vi "Launch View.vi"(8 "error in (no error)":errorcluster, 10 "ConsoleView in":refnum<class "ConsoleView.lvclass">, 11 "ConsoleInterface in":refnum<class "ConsoleSession.lvclass">) -> (0 "error out":errorcluster, 3 "ConsoleInterface out":refnum<class "ConsoleSession.lvclass">)   [LabVIEW 2019, in "ConsoleView.lvlib" / "ConsoleSession.lvclass"]
uses:
  <vilib>/gpm_packages/@cs/event-logger/Source/ConsoleView/ConsoleInterface/ConsoleSession.lvclass
  <vilib>/gpm_packages/@cs/event-logger/Source/ConsoleView/View/ConsoleView.lvclass
  <vilib>/gpm_packages/@cs/event-logger/Source/Composed Log/Types/MessageCluster.ctl
  <vilib>/gpm_packages/@cs/event-logger/Source/ConsoleView/ConsoleInterface/ConsoleSession.lvclass/ConsoleSession.ctl
  <vilib>/gpm_packages/@cs/event-logger/Source/Composed Log/Composed Log.lvlib
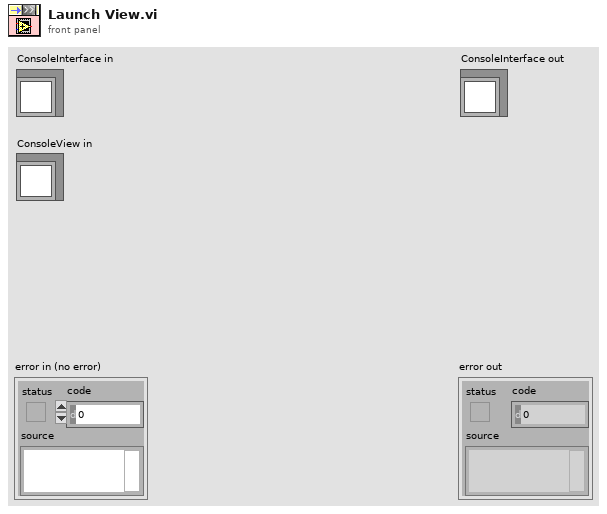
[diagram p1: front panel]
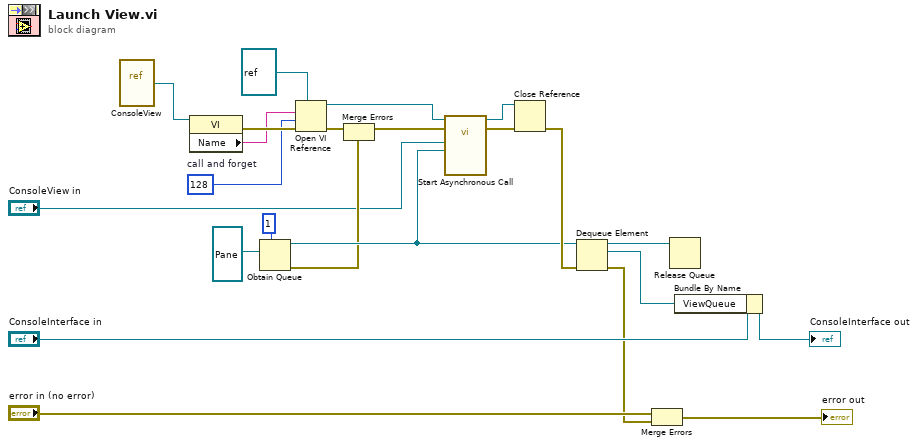
[diagram p0: block diagram]
diagram:
  w19 = 128  # call and forget
  n1 = vi-ref <vilib>:"ConsoleView.vi"() -> (w21:refnum<vi>)
  n2 = property class="VI"(reference=w21) -> (error out=w20:errorcluster, "Name"=w18:string)  [unwired: 1 in, 1 out]
  n3 = Obtain Queue(max queue size (-1, unlimited)=1, element data type=refnum<queue> refnum ("queue out")) -> (queue out=w13:refnum<queue>, error out=w10:errorcluster)  [unwired: 3 in, 1 out]
  n4 = Open VI Reference(type specifier VI Refnum (for type only)=refnum<vi> refnum, vi path=w18, options=w19, error in (no error)=w20) -> (vi reference=w8:refnum<vi>, error out=w17:errorcluster)  [unwired: 2 in]
  n5 = Merge Errors(w17, w10) -> (w11:errorcluster)
  n6 = call-by-ref "Start Asynchronous Call"(reference=w8, error in=w11, "Return Queue"=w13, "ConsoleView Sink in"="ConsoleView in") -> (reference out=w15:refnum<vi>, error out=w16:errorcluster)  [unwired: 10 in]
  n7 = Close Reference(reference=w15, error in (no error)=w16) -> (error out=w14:errorcluster)
  n8 = Dequeue Element(queue=w13, error in (no error)=w14) -> (queue out=w7:refnum<queue>, element=w5:refnum<queue>, error out=w3:errorcluster)  [unwired: 1 in, 1 out]
  n9 = Merge Errors("error in (no error)", w3) -> (→"error out":errorcluster)
  n10 = Release Queue(queue=w7) -> ()  [unwired: 2 in, 3 out]
  n11 = Bundle By Name(cluster="ConsoleInterface in", "ViewQueue"=w5) -> (→"ConsoleInterface out":refnum<class "ConsoleSession.lvclass">)
